vi "Run Measurement.vi"(6 "Show FP?":bool=TRUE, 8 "error in (no error)":errorcluster, 9 "Device Names":string[](array[string]), 10 "Measurement Name":string, 11 "Self Enqueuer In":refnum<class "Message Enqueuer.lvclass">) -> (0 "error out":errorcluster, 2 "Measurement Results":refnum<class "Results.lvclass">, 3 "Self Enqueuer Out":refnum<class "Message Enqueuer.lvclass">)   [LabVIEW 2016, in "TestStand API.lvlib"]
uses:
  TestStand API.lvlib
  <vilib>/ActorFramework/Message Enqueuer/Message Enqueuer.lvclass
  MAL-Framework/user.lib/Common Components/Results/Results.lvclass
  MAL-Framework-API/Controller API.lvclass
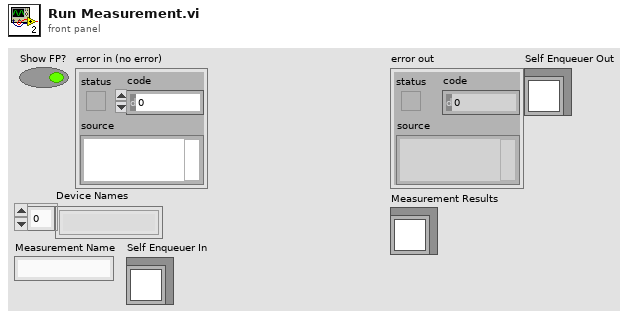
[diagram p1: front panel]
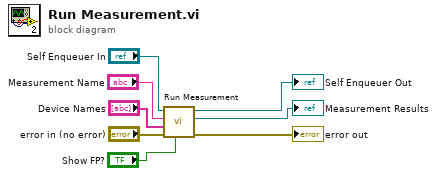
[diagram p0: block diagram]
diagram:
  n1 = call "Run Measurement.vi"("Show FP?"="Show FP?", "error in (no error)"="error in (no error)", "Device Names"="Device Names", "Measurement Name"="Measurement Name", "Self Enqueuer In"="Self Enqueuer In") -> ("error out"=→"error out":errorcluster, "Measurement Results"=→"Measurement Results":refnum<class "Results.lvclass">, "Self Enqueuer Out"=→"Self Enqueuer Out":refnum<class "Message Enqueuer.lvclass">)  [unwired: 4 in]
